vi "sine_array.vi"(6 "omega":dbl format="%#_13g", 8 "offset":dbl format="%#_13g", 9 "scale":dbl=1.0 format="%#_13g", 10 "dx":dbl=0.1 format="%#_13g", 11 "N":i32=100) -> (2 "Array":dbl[](array[numeric])=[0.0, 0.09983341664682815, 0.19866933079506122, 0.2955202066613396, 0.3894183423086505, 0.479425538604203, 0.5646424733950355, 0.6442176872376911, 0.7173560908995228, 0.7833269096274834, 0.8414709848078965, 0.8912073600614354, 0.9320390859672264, 0.963558185417193, 0.9854497299884603, 0.9974949866040544, 0.9995736030415051, 0.9916648104524686, 0.9738476308781951, 0.9463000876874145, 0.9092974268256817, 0.8632093666488737, 0.8084964038195901, 0.74570521217672, 0.6754631805511506, 0.5984721441039564, 0.5155013718214642, 0.4273798802338298, 0.33498815015590466, 0.23924932921398198, 0.1411200080598672, 0.04158066243329049, -0.058374143427580086, -0.15774569414324865, -0.25554110202683167, -0.35078322768961984, -0.44252044329485246, -0.5298361409084934, -0.6118578909427193, -0.6877661591839741, -0.7568024953079282, -0.8182771110644108, -0.8715757724135882, -0.9161659367494549, -0.951602073889516, -0.977530117665097, -0.9936910036334645, -0.9999232575641008, -0.9961646088358406, -0.9824526126243325, -0.9589242746631385, -0.9258146823277321, -0.8834546557201531, -0.8322674422239008, -0.7727644875559871, -0.7055403255703919, -0.6312666378723208, -0.5506855425976376, -0.4646021794137566, -0.373876664830236, -0.27941549819892586, -0.18216250427209502, -0.0830894028174964, 0.0168139004843506, 0.11654920485049364, 0.21511998808781552, 0.3115413635133787, 0.4048499206165983, 0.49411335113860894, 0.5784397643882001, 0.6569865987187891, 0.7289690401258765, 0.7936678638491531, 0.8504366206285648, 0.8987080958116269, 0.9379999767747389, 0.9679196720314865, 0.9881682338770004, 0.998543345374605, 0.998941341839772, 0.9893582466233818, 0.9698898108450863, 0.9407305566797726, 0.9021718337562933, 0.8545989080882804, 0.7984871126234903, 0.7343970978741133, 0.662969230082182, 0.5849171928917617, 0.5010208564578846, 0.4121184852417566, 0.3190983623493521, 0.22288991410024592, 0.1244544235070617, 0.024775425453357765, -0.0751511204618093, -0.1743267812229814, -0.2717606264109442, -0.36647912925192844, -0.45753589377532133])   [LabVIEW 2013]
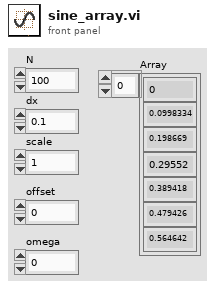
[diagram p1: front panel]
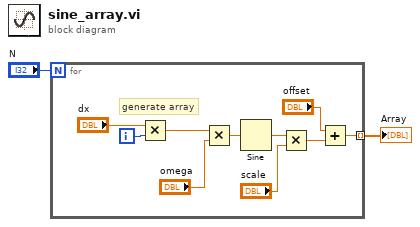
[diagram p0: block diagram]
diagram:
  n1 = for {
    N: "N" -> [_]
    tunnel: [w10] -> w1 mode=indexing
    i -> [w12]
    # "generate array"
    n2 = Multiply(x="dx", y=w12) -> (x*y=w5:dbl)
    n3 = Multiply(x=w5, y="omega") -> (x*y=w3:dbl)
    n4 = Sine(x=w3) -> (sin(x)=w7:dbl)
    n5 = Multiply(x=w7, y="scale") -> (x*y=w6:dbl)
    n6 = Add(x="offset", y=w6) -> (x+y=w10:dbl)
  }
  "Array" <- w1
